vi "REACTOR_PARSE_MIDE_PARAMETROS.vi"(11 "String":string="MEDIR Alicats 1, Temperaturas 0 , MUESTREO de 5.0s") -> (1 "Pausa (s)":dbl=1.0, 2 "Mide Alicats":bool=TRUE, 3 "Mide Eurotherm":bool=TRUE)   [LabVIEW 2017]
panel:
  # "MEDIR Alicats 1, Temperaturas 1 , MUESTREO de 5.0s"
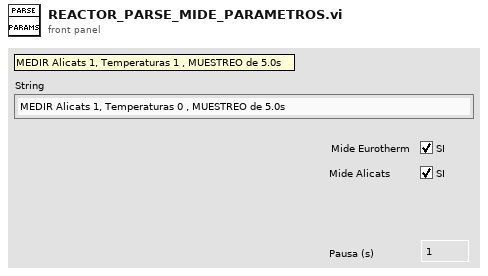
[diagram p1: front panel]
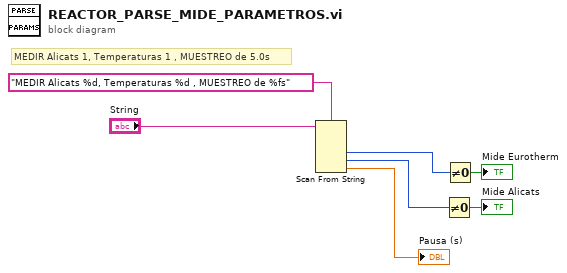
[diagram p0: block diagram]
diagram:
  # "MEDIR Alicats 1, Temperaturas 1 , MUESTREO de 5.0s"
  n1 = Scan From String(format string="MEDIR Alicats %d, Temperaturas %d , MUESTREO de %fs", input string="String") -> (output 1=w6:i32, output 2=w5:i32, output 3=→"Pausa (s)":dbl)  [unwired: 5 in, 3 out]
  n2 = Not Equal To 0?(x=w5) -> (x != 0?=→"Mide Alicats":bool)
  n3 = Not Equal To 0?(x=w6) -> (x != 0?=→"Mide Eurotherm":bool)
